vi "Markdown Library.vi"(8 "error in (no error)":errorcluster, 9 "Markdown Images Dir (..\\..\\docs\\%name%)":path=path "../../docs/api/%name%", 10 "Markdown in (..\\..\\docs\\%name%.md)":path=path "../../docs/api/%name%.md", 11 "Library Path (*.lvlib)":path=path "C:/Projects/git/LabVIEW-Queue/src/Queue.lvlib") -> (0 "error out":errorcluster, 2 "Images":path[](array[path]), 3 "Markdown out":path)   [LabVIEW 2018, in "Markdown.lvlib"]
doc: "Exports a LabVIEW Library (*.lvlib) to markdown help documentation.\n\nMarkdown template:\n\n```\n# <library_name>\n<library_description>\n\n## Examples\n<example_vi_description>\n\n## VI Tree\n<vi_tree_description>\n<palettes>\n\n## VI Descriptions\n### <VI>\n<vi_conpane_image>\n<vi_description>\n```"
uses:
  Markdown.lvlib
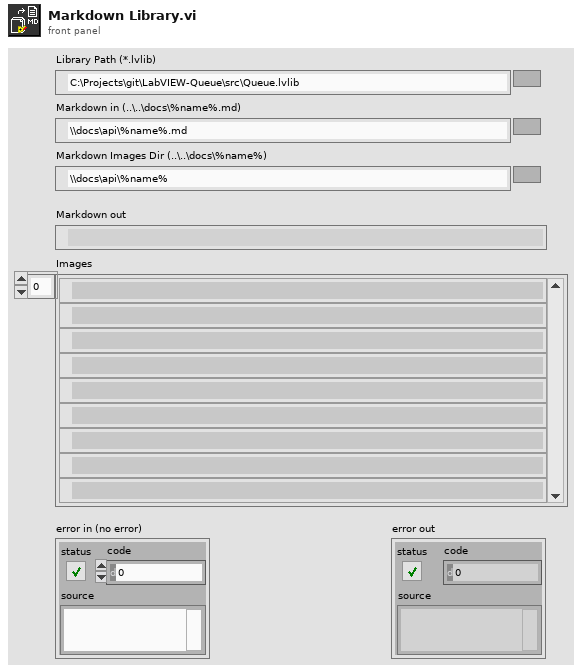
[diagram p1: front panel]
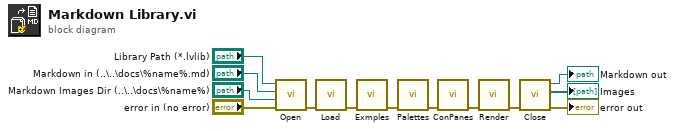
[diagram p0: block diagram]
diagram:
  n1 = call "Open.vi"("error in (no error)"="error in (no error)", "Markdown Images Dir"="Markdown Images Dir (..\\..\\docs\\%name%)", "Markdown (*.md)"="Markdown in (..\\..\\docs\\%name%.md)", "Library (*.lvlib)"="Library Path (*.lvlib)") -> ("error out"=w8:errorcluster)  [unwired: 7 in]
  n2 = call "Load.vi"("error in (no error)"=w8) -> ("error out"=w6:errorcluster)  [unwired: 10 in]
  n3 = call "Exmples.vi"("error in (no error)"=w6) -> ("error out"=w5:errorcluster)  [unwired: 10 in]
  n4 = call "Palettes.vi"("error in (no error)"=w5) -> ("error out"=w7:errorcluster)  [unwired: 10 in]
  n5 = call "ConPanes.vi"("error in (no error)"=w7) -> ("error out"=w4:errorcluster)  [unwired: 10 in]
  n6 = call "Render.vi"("error in (no error)"=w4) -> ("error out"=w3:errorcluster)  [unwired: 10 in]
  n7 = call "Close.vi"("error in (no error)"=w3) -> ("error out"=→"error out":errorcluster, "Images"=→"Images":path[], "API.md"=→"Markdown out":path)  [unwired: 8 in]
